vi "scratch-pad.vi"() -> ()   [LabVIEW 2020]
uses:
  SsaId/SsaId.lvclass
  SsaId/op_no.ctl
  SymbolRefId/SymbolRefId.lvclass
  Types/OpaqueDialectType/OpaqueDialectType.lvclass
  Operations/OpResult/OpResult.lvclass
  Operations/OpResult/count.ctl
  Types/FunctionType/FunctionType.lvclass
  Types/FloatType/FloatType.lvclass
  home/jki/Projects/mlir-labview/mlir-labview/Type/Type.lvclass
panel:
  out "mlir 6":string
  out "mlir 5":string
  out "mlir 4":string
  out "mlir 3":string
  out "mlir 2":string
  out "mlir":string
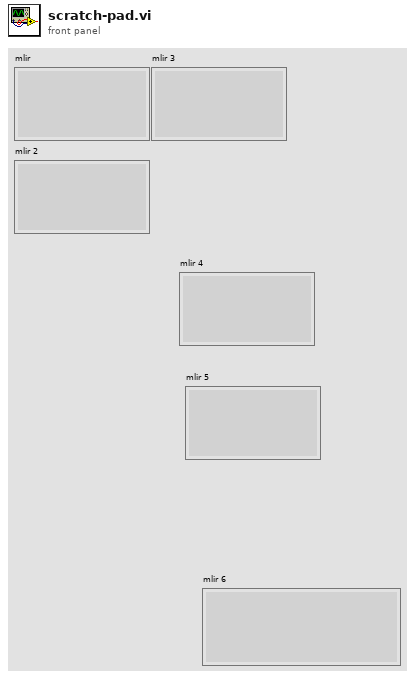
[diagram p1: front panel]
types:
  T1 = typedef "mlir.lvlib/OpResult.lvclass/count.ctl" = u32
  T2 = typedef "mlir.lvlib/SsaId.lvclass/op_no.ctl" = u32
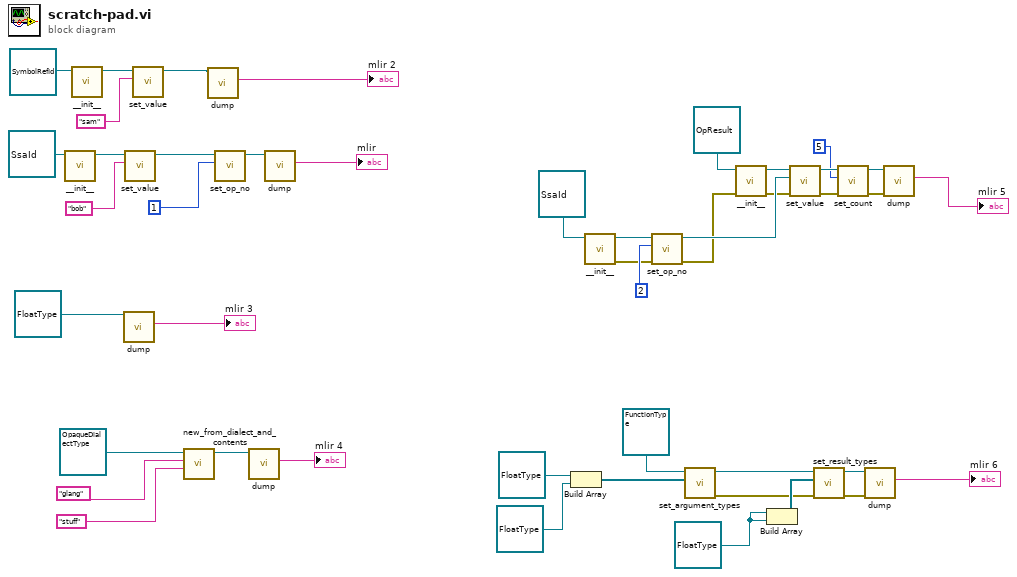
[diagram p0: block diagram]
diagram:
  w1 = refnum<class "FloatType.lvclass"> refnum ("mlir.lvlib:FloatType.lvclass")
  n1 = call-dynamic "__init__.vi"("SsaId in"=refnum<class "SsaId.lvclass"> refnum) -> ("SsaId out"=w42:refnum<class "SsaId.lvclass">)  [unwired: 9 in, 1 out]
  n2 = call-dynamic "__init__.vi"("self in"=refnum<class "SymbolRefId.lvclass"> refnum ("mlir.lvlib:SymbolRefId.lvclass")) -> ("self out"=w37:refnum<class "SymbolRefId.lvclass">)  [unwired: 9 in, 1 out]
  n3 = call-dynamic "dump.vi"("FloatType in"=refnum<class "FloatType.lvclass"> refnum ("mlir.lvlib:FloatType.lvclass")) -> ("mlir"=→"mlir 3":string)  [unwired: 8 in, 2 out]
  n4 = call-dynamic "set_value.vi"("value"="bob", "self in"=w42) -> ("self out"=w41:refnum<class "SsaId.lvclass">)  [unwired: 8 in, 1 out]
  n5 = call-dynamic "set_value.vi"("value"="sam", "self in"=w37) -> ("self out"=w35:refnum<class "SymbolRefId.lvclass">)  [unwired: 8 in, 1 out]
  n6 = call "new_from_dialect_and_contents.vi"("contents"="stuff", "dialect"="glang", "OpaqueDialectType in"=refnum<class "OpaqueDialectType.lvclass"> refnum ("mlir.lvlib:OpaqueDialectType.lvclass")) -> ("OpaqueDialectType out"=w28:refnum<class "OpaqueDialectType.lvclass">)  [unwired: 7 in, 1 out]
  n7 = call-dynamic "dump.vi"("self in"=w35) -> ("mlir"=→"mlir 2":string)  [unwired: 8 in, 2 out]
  n8 = call-dynamic "set_op_no.vi"("op_no"=T2 1, "SsaId in"=w41) -> ("SsaId out"=w40:refnum<class "SsaId.lvclass">)  [unwired: 8 in, 1 out]
  n9 = call-dynamic "dump.vi"("OpaqueDialectType in"=w28) -> ("mlir"=→"mlir 4":string)  [unwired: 8 in, 2 out]
  n10 = call-dynamic "dump.vi"("SsaId in"=w40) -> ("mlir"=→"mlir":string)  [unwired: 8 in, 2 out]
  n11 = Build Array(refnum<class "FloatType.lvclass"> refnum ("mlir.lvlib:FloatType.lvclass"), refnum<class "FloatType.lvclass"> refnum ("mlir.lvlib:FloatType.lvclass")) -> (w8:refnum<class "FloatType.lvclass">[])
  n12 = call-dynamic "__init__.vi"("SsaId in"=refnum<class "SsaId.lvclass"> refnum ("mlir.lvlib:SsaId.lvclass")) -> ("error out"=w22:errorcluster, "SsaId out"=w21:refnum<class "SsaId.lvclass">)  [unwired: 9 in]
  n13 = call-dynamic "set_op_no.vi"("error in (no error)"=w22, "op_no"=T2 2, "SsaId in"=w21) -> ("error out"=w17:errorcluster, "SsaId out"=w25:refnum<class "SsaId.lvclass">)  [unwired: 7 in]
  n14 = call-dynamic "set_argument_types.vi"("argument_types"=w8, "FunctionType in"=refnum<class "FunctionType.lvclass"> refnum ("mlir.lvlib:FunctionType.lvclass")) -> ("error out"=w5:errorcluster, "FunctionType out"=w7:refnum<class "FunctionType.lvclass">)  [unwired: 8 in]
  n15 = call-dynamic "__init__.vi"("error in (no error)"=w17, "Node in"=refnum<class "OpResult.lvclass"> refnum ("mlir.lvlib:OpResult.lvclass")) -> ("error out"=w18:errorcluster, "Node out"=w19:refnum<class "OpResult.lvclass">)  [unwired: 8 in]
  n16 = Build Array(w1, w1) -> (w6:refnum<class "FloatType.lvclass">[])
  n17 = call-dynamic "set_value.vi"("error in (no error)"=w18, "mlir.lvlib:SsaId.lvclass"=w25, "OpResult in"=w19) -> ("error out"=w14:errorcluster, "OpResult out"=w16:refnum<class "OpResult.lvclass">)  [unwired: 7 in]
  n18 = call-dynamic "set_result_types.vi"("error in (no error)"=w5, "result_types"=w6, "FunctionType in"=w7) -> ("error out"=w3:errorcluster, "FunctionType out"=w4:refnum<class "FunctionType.lvclass">)  [unwired: 7 in]
  n19 = call-dynamic "set_count.vi"("error in (no error)"=w14, "count"=T1 5, "OpResult in"=w16) -> ("error out"=w13:errorcluster, "OpResult out"=w15:refnum<class "OpResult.lvclass">)  [unwired: 7 in]
  n20 = call-dynamic "dump.vi"("error in (no error)"=w3, "FunctionType in"=w4) -> ("mlir"=→"mlir 6":string)  [unwired: 7 in, 2 out]
  n21 = call-dynamic "dump.vi"("error in (no error)"=w13, "OpResult in"=w15) -> ("mlir"=→"mlir 5":string)  [unwired: 7 in, 2 out]
